vi "GiveMeYourMediatorQueue.vi"(8 "error in (no error)":errorcluster, 10 "Reply Queue":refnum<queue>, 11 "LeakyViewModel in":refnum<class "LeakyViewModel.lvclass">) -> (0 "error out":errorcluster, 3 "LeakyViewModel out":refnum<class "LeakyViewModel.lvclass">)   [LabVIEW 2015, in "LeakyViewModel.lvlib" / "LeakyViewModel.lvclass"]
uses:
  LeakyViewModel.lvclass
  <vilib>/ActorFramework/Message Enqueuer/Message Enqueuer.lvclass
  Framework/IViewModel/IViewModel/IViewModel.lvclass/IViewModel.ctl
  Framework/IViewModel/IViewModel/IViewModel.lvclass
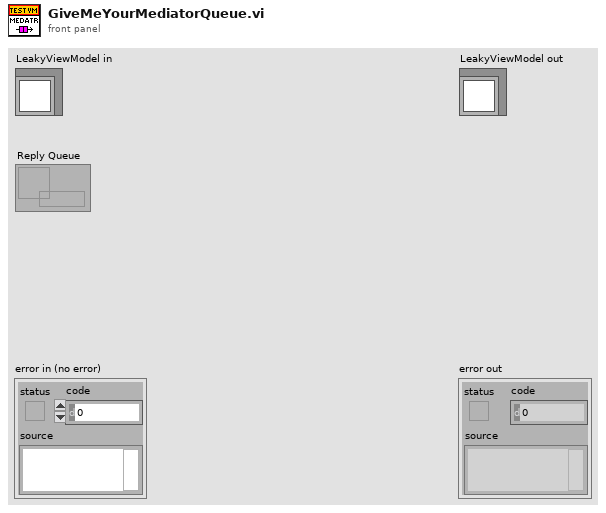
[diagram p1: front panel]
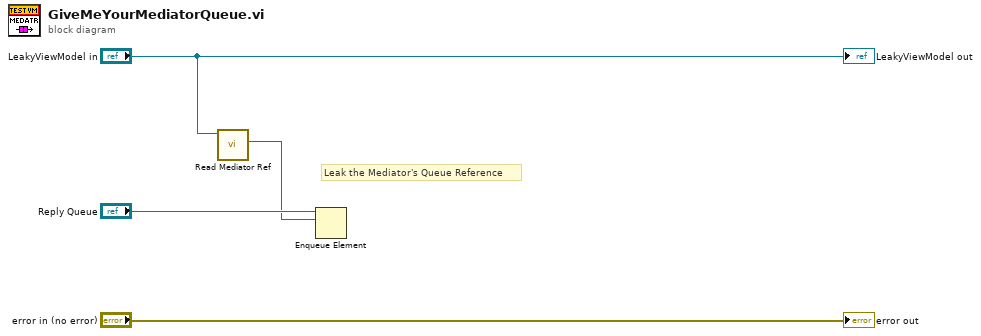
[diagram p0: block diagram]
diagram:
  # "Leak the Mediator's Queue Reference"
  n1 = call "Read Mediator Ref.vi"("IViewModel In"="LeakyViewModel in") -> ("Mediator Enququer"=w1:refnum<class "Message Enqueuer.lvclass">)  [unwired: 10 in]
  n2 = Enqueue Element(queue="Reply Queue", element=w1) -> ()  [unwired: 2 in, 3 out]
  "error out" <- "error in (no error)"
  "LeakyViewModel out" <- "LeakyViewModel in"
